vi "Simple - Runs.vi"() -> ()   [LabVIEW 2020]
uses:
  asset/asset.lvclass
  Nominal Client/Nominal Client.lvclass/Nominal Client.ctl
  Run/Run.lvclass/Run.ctl
  2308dcb4-1185-4fbb-9f93-c47e786e00a6.vi
  Run/runNumber.get.vi
  Run/asset.get.vi
  Run/assets.get.vi
  Run/attachments.get.vi
  Run/authorRid.get.vi
  Run/createdAt.get.vi
  Nominal Client/private_data.set.vi
  Run/asset.get.vi/de85e14f-50dd-4ec2-a9b0-0cc4386a757e.vi
  Run/assets.get.vi/fc990382-c15b-405e-8523-435b97eca7cf.vi
  Run/attachments.get.vi/f8940fc2-285b-4416-aebd-2c1d34bf7d3c.vi
  Run/authorRid.get.vi/00467254-ce2c-4e37-b69b-d84d91206466.vi
  Nominal Client/iso8601_string_to_timestamp.vi
  Run/createdAt.get.vi/b3b51881-3115-4bdb-b91c-b9f37aeec093.vi
  Run/asset.get.vi/de85e14f-50dd-4ec2-a9b0-0cc4386a757e.vi/32c3acc2-0975-485a-8283-62feb0f3dc4f.vi
  Run/run_properties.get.vi
  Run/assets.get.vi/fc990382-c15b-405e-8523-435b97eca7cf.vi/32c3acc2-0975-485a-8283-62feb0f3dc4f.vi
  Run/attachments.get.vi/f8940fc2-285b-4416-aebd-2c1d34bf7d3c.vi/32c3acc2-0975-485a-8283-62feb0f3dc4f.vi
  Run/authorRid.get.vi/00467254-ce2c-4e37-b69b-d84d91206466.vi/32c3acc2-0975-485a-8283-62feb0f3dc4f.vi
  Run/createdAt.get.vi/b3b51881-3115-4bdb-b91c-b9f37aeec093.vi/32c3acc2-0975-485a-8283-62feb0f3dc4f.vi
  <vilib>/Utility/file.llb/Application Directory.vi
  <vilib>/Utility/error.llb/Error Cluster From Error Code.vi
  submodules/reqwest-labview/lv-src/reqwest/create.vi
  Run/update.cache.vi
  <vilib>/JDP Science/JSONtext/JSON type.vi
  <vilib>/JDP Science/JSONtext/JSON text to Variant.vi
  Nominal Client/asset.get.vi
  Nominal Client/asset.get[].vi
  <vilib>/LabVIEW Open Source Project/Epoch Date & Time/formatter.iso8601/ISO8601 DateString to Timestamp.vi
  Nominal Client/Nominal Client.lvclass
  nominal types/workspace/workspace.lvclass
  submodules/reqwest-labview/lv-src/reqwest/reqwest.lvclass
  <vilib>/JDP Science/JSONtext/LVClass Serializer/JSONtext LVClass Serializer.lvclass
  Run/Run.lvclass
panel:
  in  "Assets":refnum<class "asset.lvclass">[](array[class])
  in  "Description":string
  in  "End Time (now)":timestamp format="%<%x %.3X>T"
  in  "labels":string[](array[string])
  in  "Links":map{string, string}(c390)
  in  "Updated Title":string
  in  "properties":map{string, string}(c390)
  in  "Start Time (now)":timestamp format="%<%x %.3X>T"
  in  "Title":string
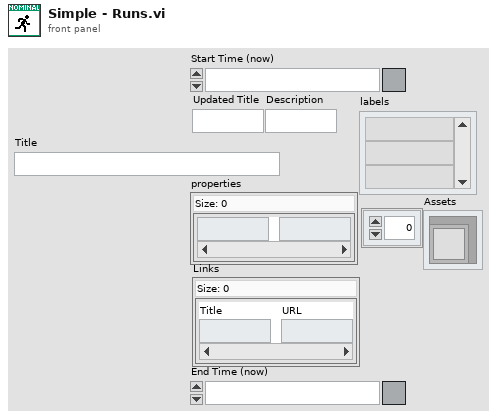
[diagram p1: front panel]
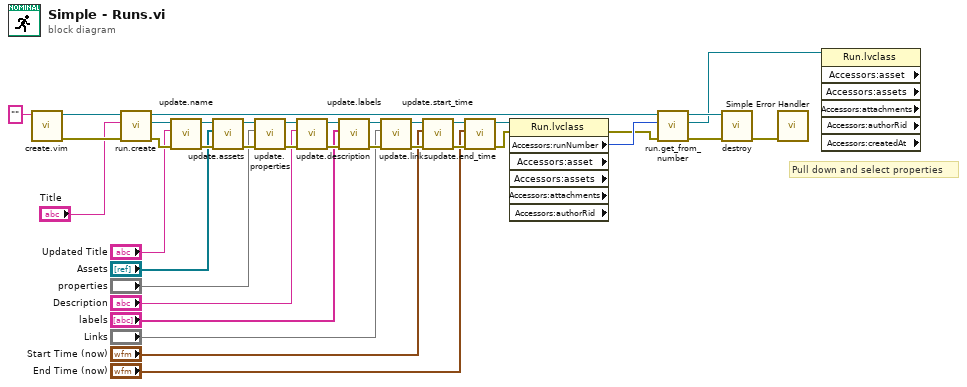
[diagram p0: block diagram]
diagram:
  # "Pull down and select properties"
  n1 = call "create.vim"("API Token (string or path)"="") -> ("error out"=w34:errorcluster, "Nominal Client"=w35:refnum<class "Nominal Client.lvclass">)  [unwired: 9 in]
  n2 = call "run.create.vi"("error in"=w34, "Title"="Title", "Nominal Client in"=w35) -> ("error out"=w10:errorcluster, "Run"=w29:refnum<class "Run.lvclass">, "Nominal Client out"=w11:refnum<class "Nominal Client.lvclass">)  [unwired: 6 in]
  n3 = call "update.name.vi"("error in (no error)"=w10, "Title"="Updated Title", "Run in"=w29) -> ("error out"=w27:errorcluster, "Run out"=w28:refnum<class "Run.lvclass">)  [unwired: 7 in]
  n4 = call "update.assets.vi"("error in (no error)"=w27, "Assets"="Assets", "Run in"=w28) -> ("error out"=w25:errorcluster, "Run out"=w26:refnum<class "Run.lvclass">)  [unwired: 7 in]
  n5 = call "update.properties.vi"("error in (no error)"=w25, "properties"="properties", "Run in"=w26) -> ("error out"=w23:errorcluster, "Run out"=w24:refnum<class "Run.lvclass">)  [unwired: 7 in]
  n6 = call "update.description.vi"("error in (no error)"=w23, "Description"="Description", "Run in"=w24) -> ("error out"=w21:errorcluster, "Run out"=w22:refnum<class "Run.lvclass">)  [unwired: 7 in]
  n7 = call "update.labels.vi"("error in (no error)"=w21, "labels"="labels", "Run in"=w22) -> ("error out"=w19:errorcluster, "Run out"=w20:refnum<class "Run.lvclass">)  [unwired: 7 in]
  n8 = call "update.links.vi"("error in (no error)"=w19, "Links"="Links", "Run in"=w20) -> ("error out"=w17:errorcluster, "Run out"=w18:refnum<class "Run.lvclass">)  [unwired: 7 in]
  n9 = call "update.start_time.vi"("error in (no error)"=w17, "Start Time (now)"="Start Time (now)", "Run in"=w18) -> ("error out"=w15:errorcluster, "Run out"=w16:refnum<class "Run.lvclass">)  [unwired: 7 in]
  n10 = call "update.end_time.vi"("error in (no error)"=w15, "End Time (now)"="End Time (now)", "Run in"=w16) -> ("error out"=w12:errorcluster, "Run out"=w14:refnum<class "Run.lvclass">)  [unwired: 7 in]
  n11 = property class="Run.lvclass" props=["Accessors:runNumber", "Accessors:asset", "Accessors:assets", "Accessors:attachments", "Accessors:authorRid"](reference=w14, error in=w12) -> (error out=w13:errorcluster, "Accessors:runNumber"=w31:i32)  [unwired: 5 out]
  n12 = call "run.get_from_number.vi"("error in"=w13, "Run Number"=w31, "Nominal Client in"=w11) -> ("error out"=w32:errorcluster, "Run"=w9:refnum<class "Run.lvclass">, "Nominal Client out"=w33:refnum<class "Nominal Client.lvclass">)  [unwired: 6 in]
  n13 = call "destroy.vi"("error in"=w32, "Nominal Client"=w33) -> ("error out"=w36:errorcluster)  [unwired: 9 in]
  n14 = call <vilib>:"Simple Error Handler.vi"("error in (no error)"=w36) -> ()  [unwired: 4 in, 5 out]
  n15 = property class="Run.lvclass" props=["Accessors:asset", "Accessors:assets", "Accessors:attachments", "Accessors:authorRid", "Accessors:createdAt"](reference=w9) -> ()  [unwired: 1 in, 7 out]
